vi "Overlay Features.vi"(8 "error in (no error)":errorcluster, 10 "Features":T1[](array[typedef]), 11 "Refnum in":T2) -> (0 "Error Out":errorcluster, 3 "Refnum out":T2)   [LabVIEW 2022 SP3, in "Coin Analyser.lvclass"]
uses:
  <vilib>/vision/Image Controls.llb/IMAQ Image.ctl
  Coins.ctl
  Coin Analyser.lvclass
  Coin Analyser.lvclass/Coin Analyser.ctl
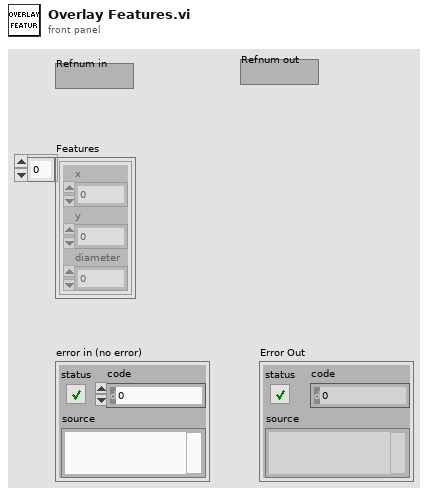
[diagram p1: front panel]
types:
  T1 = typedef "Coin Analyser.lvclass/Coins.ctl" = cluster{"x":i32, "y":i32, "diameter":i32}
  T2 = typedef "IMAQ Image.ctl" = refnum<image>
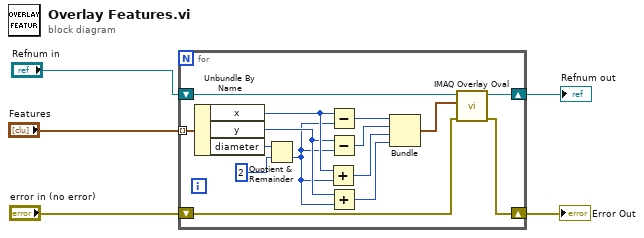
[diagram p0: block diagram]
diagram:
  n1 = for {
    tunnel: "Features" -> [w19] mode=indexing
    shift-right: [w10] -> w4
    shift-left: "Refnum in" -> [w20]
    shift-right: [w6] -> w1
    shift-left: "error in (no error)" -> [w7]
    n2 = Unbundle By Name(w19) -> ("x"=w18:i32, "y"=w17:i32, "diameter"=w16:i32)
    n3 = Quotient & Remainder(x=w16, y=2) -> (floor(x/y)=w8:i32)  [unwired: 1 out]
    n4 = Add(x=w18, y=w8) -> (x+y=w13:i32)
    n5 = Subtract(x=w18, y=w8) -> (x-y=w15:i32)
    n6 = Subtract(x=w17, y=w8) -> (x-y=w14:i32)
    n7 = Add(x=w17, y=w8) -> (x+y=w12:i32)
    n8 = Bundle(w15, w14, w13, w12) -> (w11:cluster{i32, i32, i32, i32})  [unwired: 1 in]
    n9 = call "IMAQ Overlay Oval"("error in (no error)"=w7, "Bounding Rectangle"=w11, "Image"=w20) -> ("error out"=w6:errorcluster, "Image Out"=w10:T2)  [unwired: 7 in]
  }
  "Refnum out" <- w4
  "Error Out" <- w1
